vi "connect_two_terminal.vi"(8 "error in":errorcluster, 9 "Auto Route? (T)":bool=TRUE, 10 "Terminal 2":refnum<vi>, 11 "Terminal 1":refnum<vi>) -> (0 "error out":errorcluster)   [LabVIEW 2018]
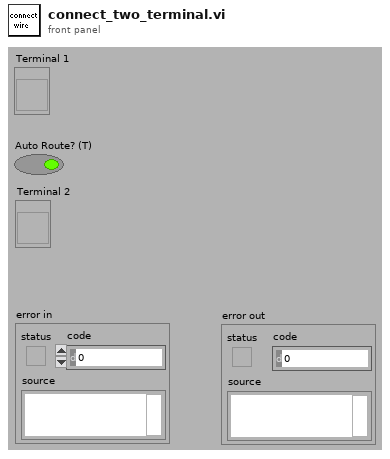
[diagram p1: front panel]
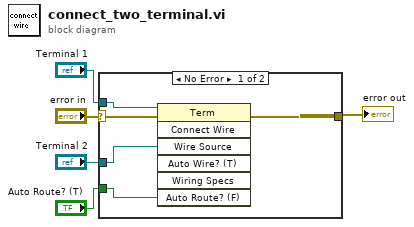
[diagram p0: block diagram]
diagram:
  n1 = case shown="No Error" "error in" {
    selector: "error in" -> [w8 w11]
    tunnel: [w6 w11] -> w5
    tunnel: "Terminal 2" -> [w7 _]
    tunnel: "Auto Route? (T)" -> [w10 _]
    tunnel: "Terminal 1" -> [w9 _]
    frame No Error {
      n2 = invoke class="Term" method="Connect Wire"(reference=w9, error in=w8, "Wire Source"=w7, "Auto Route? (F)"=w10) -> (error out=w6:errorcluster)  [unwired: 3 in, 6 out]
    }
    frame Error {
    }
  }
  "error out" <- w5
